vi "Initialize Tree.vi"(8 "error in (no error)":errorcluster, 11 "Application Data in":T1) -> (0 "error out":errorcluster, 1 "async plugins tag":string, 2 "inline plugins tag":string, 3 "Application Data out":T1)   [LabVIEW 2017, in "DSF Data Viewer.lvlib"]
uses:
  DSF Data Viewer.lvlib
  Application Data.ctl
  Builds/Data Sharing Framework/Current/Core/DSF Core.lvlibp/Engine/Classes/Framework/Framework.lvclass
  <vilib>/NI/Memory Manager/Classes/Pointer/Pointer.lvclass
  Buffer Reader/Buffer Data.ctl
  Builds/Data Sharing Framework/Current/Core/DSF Core.lvlibp/Engine/Classes/Buffer/Buffer.lvclass
  Item Tree/Create New Tree Item.vi
  Item Tree/Add Buffer Data to Variant.vi
  Item Tree/Add Item to Tree.vi
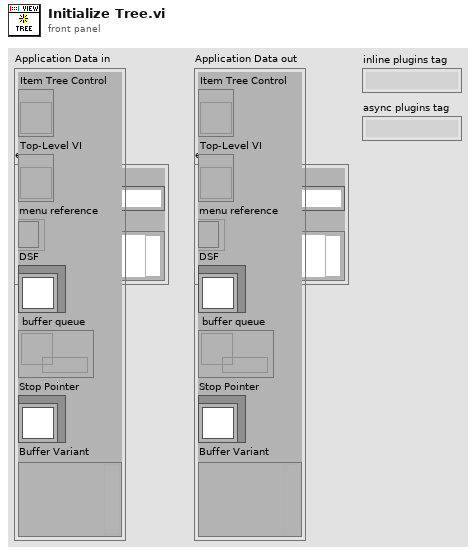
[diagram p1: front panel]
types:
  T1 = typedef "DSF Data Viewer.lvlib/Application Data.ctl" = cluster{"Item Tree Control":refnum<vi>, "Top-Level VI":refnum<vi>, "menu reference":refnum<k9>, "DSF":refnum<class "Framework.lvclass">, "buffer queue":refnum<queue>, "Stop Pointer":refnum<class "Pointer.lvclass">, "Buffer Variant":variant}
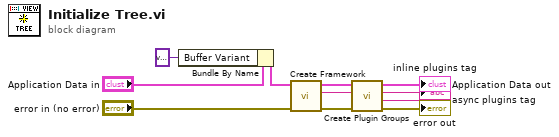
[diagram p0: block diagram]
diagram:
  n1 = Bundle By Name(cluster="Application Data in", "Buffer Variant"=variant) -> (w9:T1)
  n2 = call "Create Framework.vi"("error in (no error)"="error in (no error)", "Application Data in"=w9) -> ("error out"=w6:errorcluster, "new item tag"=w5:string, "Application Data Out"=w7:T1)  [unwired: 7 in]
  n3 = call "Create Plugin Groups.vi"("error in (no error)"=w6, "parent tag"=w5, "Application Data In"=w7) -> ("error out"=→"error out":errorcluster, "async plugins tag"=→"async plugins tag":string, "inline plugins tag"=→"inline plugins tag":string, "Application Data out"=→"Application Data out":T1)  [unwired: 5 in]
